vi "Configure Slew Mode.vi"(7 "Channel (0: Channel A)":u16(ring) items=["Channel A", "Channel B"], 8 "error in (no error)":errorcluster, 10 "Slew Mode (Maximum)":string(combo)="max", 11 "BH Druck PACE Series in":refnum<class "BH Druck PACE Series.lvclass">) -> (0 "error out":errorcluster, 3 "BH Druck PACE Series out":refnum<class "BH Druck PACE Series.lvclass">)   [LabVIEW 2022 SP3, in "BH Druck PACE Series.lvclass"]
uses:
  BH Druck PACE Series.lvclass
  BH Druck PACE Series.lvclass/BH Druck PACE Series.ctl
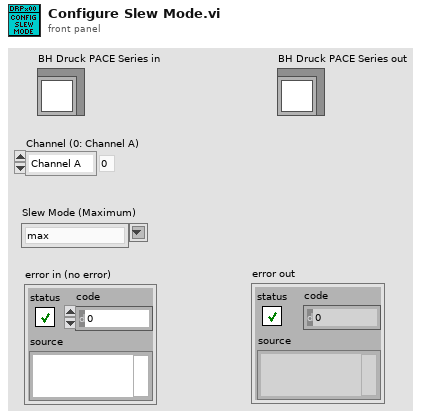
[diagram p1: front panel]
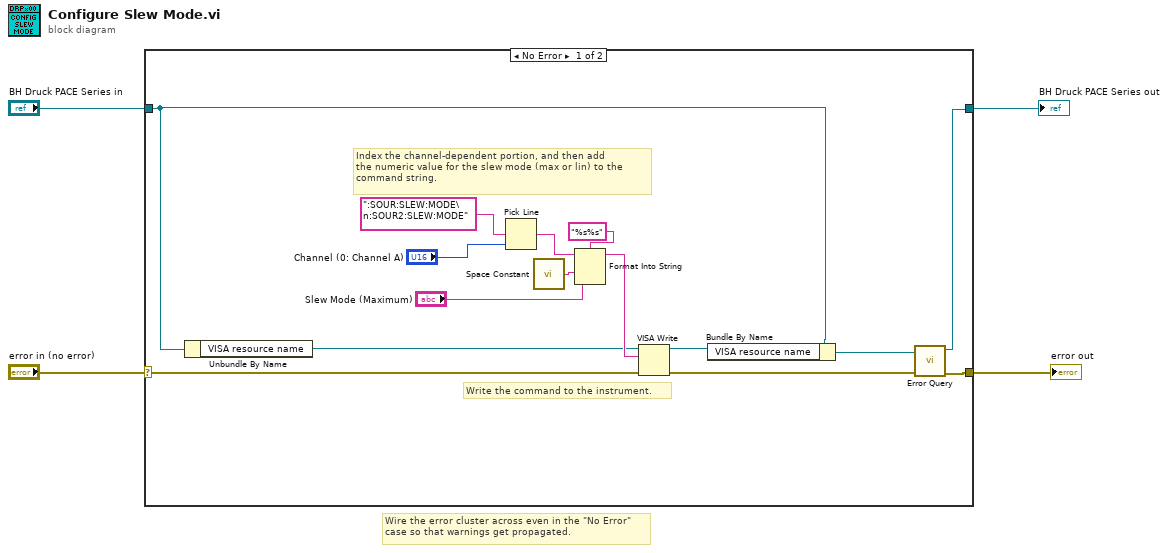
[diagram p0: block diagram]
diagram:
  # "Wire the error cluster across even in the \"No Error\"\ncase so that warnings get propagated."
  n1 = case shown="No Error" "error in (no error)" {
    selector: "error in (no error)" -> [w12 w21]
    tunnel: [w10 w21] -> w3
    tunnel: [w5 w20] -> w1
    tunnel: "BH Druck PACE Series in" -> [w9 w20]
    frame No Error {
      # "Index the channel-dependent portion, and then add\nthe numeric value for the slew mode (max or lin) to the \ncommand string."
      # "Write the command to the instrument."
      n2 = Unbundle By Name(w9) -> ("VISA resource name"=w11:refnum<visa-resource-name>)
      n3 = Pick Line(multi-line string=":SOUR:SLEW:MODE\n:SOUR2:SLEW:MODE", line index="Channel (0: Channel A)") -> (output string=w19:string)  [unwired: 1 in]
      n4 = call <vilib>:"Space Constant.vi"() -> ("String"=w17:string)
      n5 = Format Into String(format string="%s%s", initial string=w19, w17, "Slew Mode (Maximum)") -> (resulting string=w16:string)  [unwired: 1 in, 1 out]
      n6 = VISA Write(VISA resource name=w11, write buffer=w16, error in (no error)=w12) -> (VISA resource name out=w8:refnum<visa-resource-name>, error out=w6:errorcluster)  [unwired: 1 out]
      n7 = Bundle By Name(cluster=w9, "VISA resource name"=w8) -> (w7:refnum<class "BH Druck PACE Series.lvclass">)
      n8 = call-dynamic "Error Query.vi"("error in (no error)"=w6, "BH Druck PACE Series in"=w7) -> ("error out"=w10:errorcluster, "BH Druck PACE Series out"=w5:refnum<class "BH Druck PACE Series.lvclass">)  [unwired: 8 in]
    }
    frame Error {
    }
  }
  "error out" <- w3
  "BH Druck PACE Series out" <- w1
